vi "set_communications_configuration.vi"(6 "Echo on":bool=TRUE, 8 "error in (no error)":errorcluster, 9 "Comms":string(combo)="330", 10 "Comms configuration cluster":T1={"Protocol"="0", "Data mode"="0", "Line feed enabled"="0", "Response echo enabled"="0", "Separation char (Omega protocol, continuous data mode)"="0"}, 11 "connection ID":refnum<k5>) -> (0 "error out":errorcluster, 3 "connection ID out":refnum<k5>)   [LabVIEW 2018]
uses:
  typedefs/communications_configuration.ctl
panel:
  out "Response":string
  in  "Separation char (Omega protocol, continuous data mode)":string(combo)="0"
  in  "Response echo enabled":string(combo)="0"
  in  "Line feed enabled":string(combo)="0"
  in  "Data mode":string(combo)="0"
  in  "Protocol":string(combo)="0"
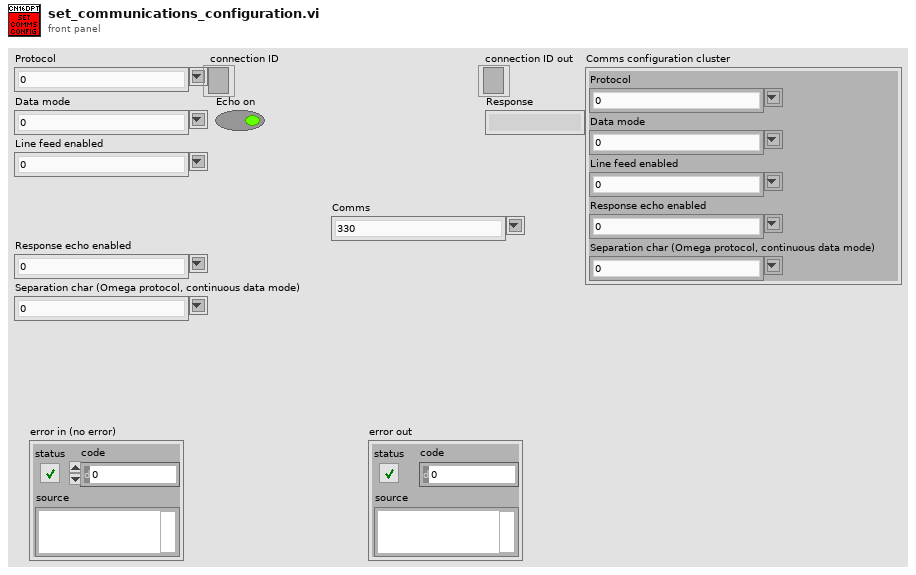
[diagram p1: front panel]
types:
  T1 = typedef "communications_configuration.ctl" = cluster{"Protocol":string, "Data mode":string, "Line feed enabled":string, "Response echo enabled":string, "Separation char (Omega protocol, continuous data mode)":string}
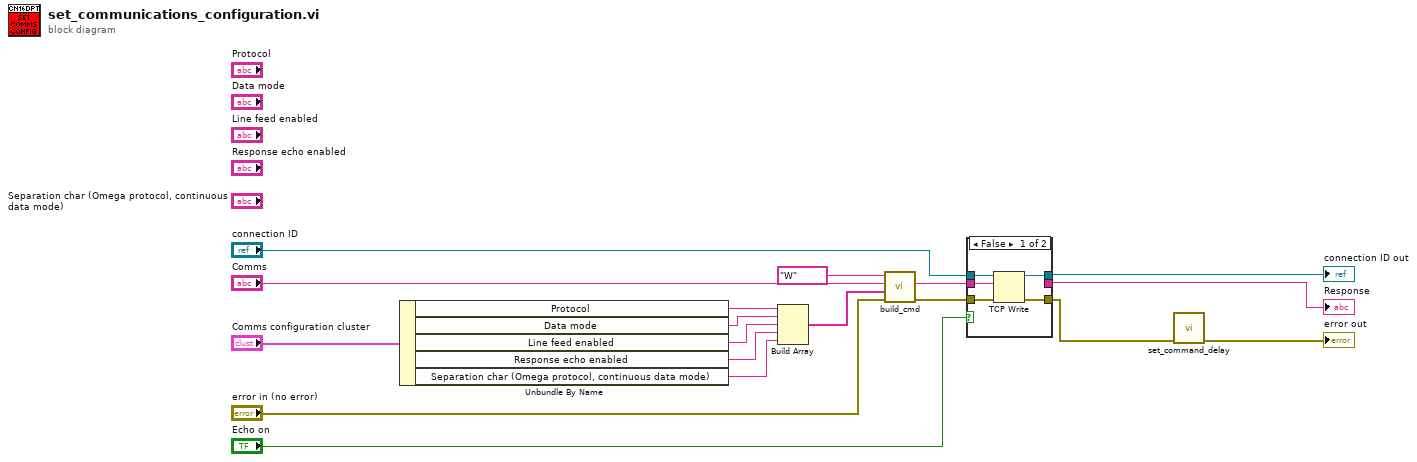
[diagram p0: block diagram]
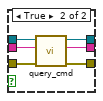
[diagram p2: hidden frame]
diagram:
  n1 = Unbundle By Name("Comms configuration cluster") -> ("Protocol"=w8:string, "Data mode"=w7:string, "Line feed enabled"=w6:string, "Response echo enabled"=w5:string, "Separation char (Omega protocol, continuous data mode)"=w4:string)
  n2 = Build Array(w8, w7, w6, w5, w4) -> (w17:string[])
  n3 = call "build_cmd.vi"("error in (no error)"="error in (no error)", "Parameter list"=w17, "Command ID"="Comms", "Command class"="W") -> ("error out"=w15:errorcluster, "Command"=w14:string)  [unwired: 6 in]
  n4 = case shown="False" "Echo on" {
    tunnel: [w21 w29] -> w2
    tunnel: w15 -> [w22 w28]
    tunnel: w14 -> [w19 w27]
    tunnel: [w20 w26] -> w12
    tunnel: "connection ID" -> [w23 w25]
    tunnel: [_ w24] -> w10
    frame False {
      n5 = TCP Write(connection ID=w23, data in=w19, error in (no error)=w22) -> (connection ID out=w20:refnum<k5>, error out=w21:errorcluster)  [unwired: 1 in, 1 out]
    }
    frame True {
      n6 = call "query_cmd.vi"("error in (no error)"=w28, "Command"=w27, "connection ID"=w25) -> ("error out"=w29:errorcluster, "Response"=w24:string, "connection ID out"=w26:refnum<k5>)  [unwired: 6 in]
    }
  }
  "connection ID out" <- w12
  "Response" <- w10
  n7 = call "set_command_delay.vi"("error in (no error)"=w2) -> ("error out"=→"error out":errorcluster)  [unwired: 10 in]
